vi "Player Info.vi"(8 "Victory Speech":string="Got Hunger?", 9 "Name":string="Hungry Wolf", 11 "Hungry Wolf in":refnum<class "Hungry Wolf.lvclass">) -> (3 "Hungry Wolf out":refnum<class "Hungry Wolf.lvclass">)   [LabVIEW 2015, in "Hungry Wolf.lvclass"]
uses:
  Hungry Wolf.lvclass
  Square/Square.lvclass
panel:
  # "Set default values for these two string controls"
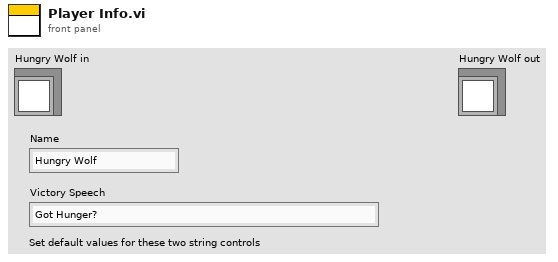
[diagram p1: front panel]
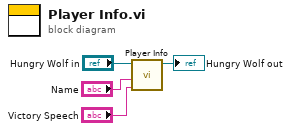
[diagram p0: block diagram]
diagram:
  n1 = call-parent "Player Info.vi"("Victory Speech"="Victory Speech", "Name"="Name", "Square in"="Hungry Wolf in") -> ("Square out"=→"Hungry Wolf out":refnum<class "Hungry Wolf.lvclass">)  [unwired: 8 in]
